vi "init.vi"(8 "error in (no error)":errorcluster, 11 "ITaskStopMechanism in":refnum<class "ITaskChannel.lvclass">) -> (0 "error out":errorcluster, 3 "ITaskStopMechanism out":refnum<class "ITaskChannel.lvclass">)   [LabVIEW 2023, in "TLC_Daemon.lvlib" / "ITaskChannel.lvclass"]
doc: "Initializes the Task Channel."
uses:
  ITaskChannel.lvclass
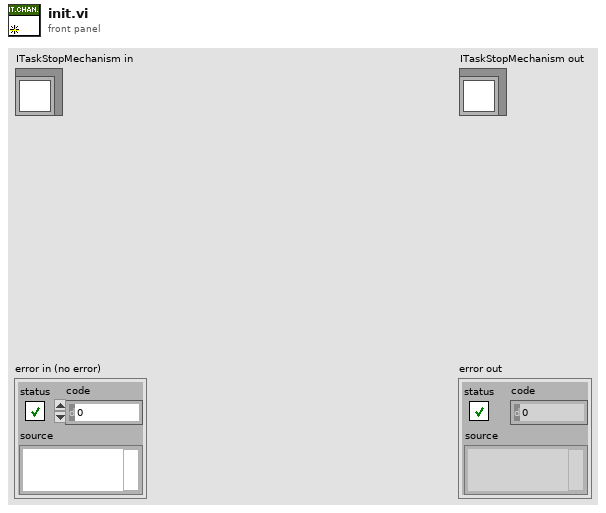
[diagram p1: front panel]
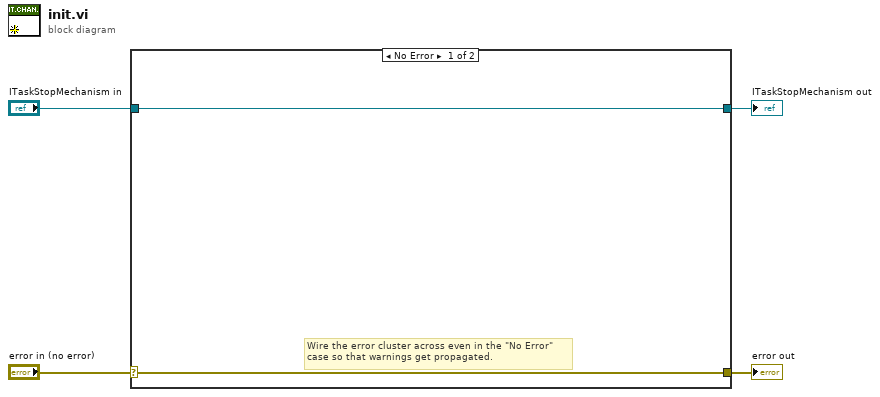
[diagram p0: block diagram]
diagram:
  n1 = case shown="No Error" "error in (no error)" {
    selector: "error in (no error)" -> [w5 w8]
    tunnel: [w5 w8] -> w3
    tunnel: [w6 w7] -> w1
    tunnel: "ITaskStopMechanism in" -> [w6 w7]
    frame No Error {
      # "Wire the error cluster across even in the \"No Error\"\ncase so that warnings get propagated."
    }
    frame Error {
    }
  }
  "error out" <- w3
  "ITaskStopMechanism out" <- w1
